vi "Set Page Size.vi"(0 "PDF Report IN":refnum<class "PDF Report Class.lvclass">, 2 "Page setup":T1={"Page Size"=1, "Orientation"=enum."Portrait", "Custom Size"={"Width"=0.0, "Height"=0.0}, "Margins"={"Left"=25.0, "Right"=25.0, "Top"=25.0, "Bottom"=25.0}} {"Page Size" items=["Custom", "LETTER", "NOTE", "LEGAL", "TABLOID", "EXECUTIVE", "POSTCARD", "A0", "A1", "A2", "A3", "A4", "A5", "A6", "A7", "A8", "A9", "A10", "B0", "B1", "B2", "B3", "B4", "B5", "B6", "B7", "B8", "B9", "B10", "ARCH_E", "ARCH_D", "ARCH_C", "ARCH_B", "ARCH_A", "FLSA", "FLSE", "HALFLETTER", "_11X17", "ID_1", "ID_2", "ID_3", "LEDGER", "CROWN_QUARTO", "LARGE_CROWN_QUARTO", "DEMY_QUARTO", "ROYAL_QUARTO", "CROWN_OCTAVO", "LARGE_CROWN_OCTAVO", "DEMY_OCTAVO", "ROYAL_OCTAVO", "SMALL_PAPERBACK", "PENGUIN_SMALL_PAPERBACK", "PENGUIN_LARGE_PAPERBACK"]}, 11 "error in (no error)":errorcluster) -> (4 "PDF Report OUT":refnum<class "PDF Report Class.lvclass">, 15 "error OUT":errorcluster)   [LabVIEW 2019]
doc: "Creates a page break within the PDF report and change the layout of the new page:\n- Page size;\n- Orientation;\n- Margins (mm or in);\n- Custom layout (if Page size = custom, mm or in);\n\nMinimum page size: 3 points x 3 points (1.06 mm x 1.06 mm or 0.042 in x 0.042 in)\nMaximum page size: 14400 points x 14400 points (5.08 m x 5.08 m or 200 in x 200 in)\n\n<B>FRANÇAIS</B>\nAjoute un saut de page dans le rapport PDF et change les caractéristiques de la nouvelle page :\n- Format de la page;\n- Orientation;\n- Marges (mm or in);\n- Format personnalisé (si Page size = custom, mm ou in).\n\nDimensions minimales d'une page: 3 points x 3 points (1.06 mm x 1.06 mm or 0.042 in x 0.042 in).\nDimensions maximales d'une page: 14400 points x 14400 points (5.08 m x 5.08 m or 200 in x 200 in).\n\nVersion 1.0\nDeveloped by Jean-Marc Simard\nCopyright © 2010, Exaprom Inc.\nAll rights reserved.\nLicense: BSD\n\nWith iTextSharp 4.1.6 (http://itextsharp.sourceforge.net)\nunder Mozilla Public License Version 1.1\n(http://www.mozilla.org/MPL/MPL-1.1.html)"
uses:
  <userlib>/Exaprom PDF/Controls/Page Controls/Page setup.ctl
  <userlib>/Exaprom PDF/Controls/Page Controls/Page size.ctl
  <userlib>/Exaprom PDF/Controls/Page Controls/Page Orientation.ctl
  <userlib>/Exaprom PDF/Controls/Page Controls/Page Layout Custom.ctl
  <userlib>/Exaprom PDF/Controls/Page Controls/Page margins.ctl
  <userlib>/Exaprom PDF/LV Class/PDF Report Class/PDF Report Class.lvclass
  C:/Program Files/National Instruments/LabVIEW 2019/user.lib/Exaprom PDF/DLL/itextsharp.dll
  DLL/itextsharp.dll
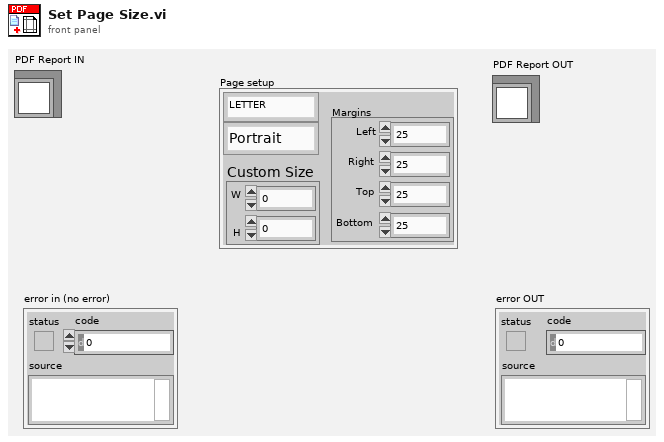
[diagram p1: front panel]
types:
  T1 = typedef "Page setup.ctl" = cluster{"Page Size":T2, "Orientation":T3, "Custom Size":T4, "Margins":T5}
  T2 = typedef "Page size.ctl" = i32
  T3 = typedef "Page Orientation.ctl" = enum16{"Portrait", "Landscape"}
  T4 = typedef "Page Layout Custom.ctl" = cluster{"Width":sgl, "Height":sgl}
  T5 = typedef "Page margins.ctl" = cluster{"Left":sgl, "Right":sgl, "Top":sgl, "Bottom":sgl}
  T6 = typedef "Page dimensions.ctl" = cluster{"Start at page":i32, "Page Size":T2, "Orientation":T3, "widht":sgl, "height":sgl, "Margin left":sgl, "Margin right":sgl, "Margin top":sgl, "Margin bottom":sgl, "X0":sgl, "X1":sgl, "Y0":sgl, "Y1":sgl}
  T7 = typedef "Unit.ctl" = enum16{"inch", "mm"}
  T8 = cluster{"PageNumber":i32, "Page Size":T2, "Orientation":T3, "Width":sgl, "Height":sgl, "LeftMargin":sgl, "RightMargin":sgl, "TopMargin":sgl, "BottomMargin":sgl, "widht":sgl, "Width":sgl, "widht":sgl, "Height":sgl}
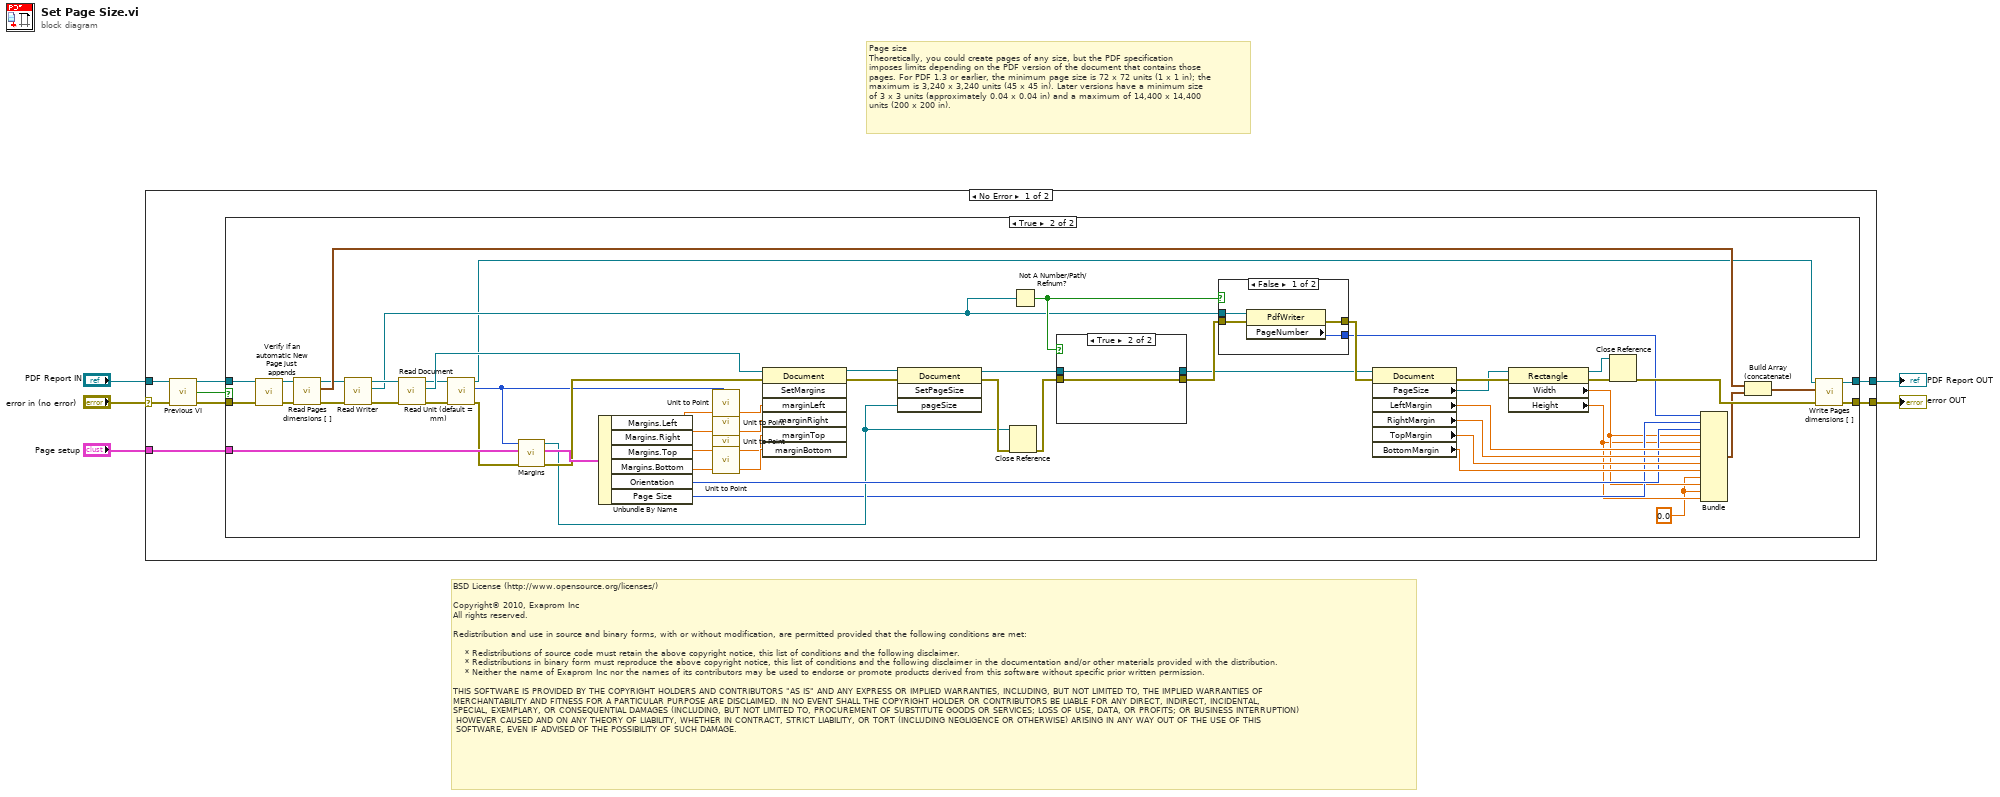
[diagram p0: block diagram]
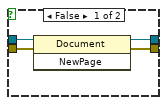
[diagram p3: hidden frame]
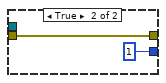
[diagram p4: hidden frame]
diagram:
  # "Page size\nTheoretically, you could create pages of any size, but the PDF specification\nimposes limits depending on the PDF version of the document that contains those\npages. For PDF 1.3 or earlier, the minimum page size is 72 x 72 units (1 x 1 in); the\nmaximum is 3,240 x 3,240 units (45 x 45 in). Later versions have a minimum size\nof 3 x 3 units (approximately 0.04 x 0.04 in) and a maximum of 14,400 x 14,400\nunits (200 x 200 in)."
  # "BSD License (http://www.opensource.org/licenses/)\n\nCopyright© 2010, Exaprom Inc\nAll rights reserved.\n\nRedistribution and use in source and binary forms, with or without modification, are permitted provided that the following conditions are met:\n\n    * Redistributions of source code must retain the above copyright notice, this list of conditions and the following disclaimer.\n    * Redistributions in binary form must reproduce the above copyright notice, this list of conditions and the following disclaimer in the documentation and/or other materials provided with the distribution.\n    * Neither the name of Exaprom Inc nor the names of its contributors may be used to endorse or promote products derived from this software without specific prior written permission.\n\nTHIS SOFTWARE IS PROVIDED BY THE COPYRIGHT HOLDERS AND CONTRIBUTORS \"AS IS\" AND ANY EXPRESS OR IMPLIED WARRANTIES, INCLUDING, BUT NOT LIMITED TO, THE IMPLIED WARRANTIES OF \nMERCHANTABILITY AND FITNESS FOR A PARTICULAR PURPOSE ARE DISCLAIMED. IN NO EVENT SHALL THE COPYRIGHT HOLDER OR CONTRIBUTORS BE LIABLE FOR ANY DIRECT, INDIRECT, INCIDENTAL,\nSPECIAL, EXEMPLARY, OR CONSEQUENTIAL DAMAGES (INCLUDING, BUT NOT LIMITED TO, PROCUREMENT OF SUBSTITUTE GOODS OR SERVICES; LOSS OF USE, DATA, OR PROFITS; OR BUSINESS INTERRUPTION)\n HOWEVER CAUSED AND ON ANY THEORY OF LIABILITY, WHETHER IN CONTRACT, STRICT LIABILITY, OR TORT (INCLUDING NEGLIGENCE OR OTHERWISE) ARISING IN ANY WAY OUT OF THE USE OF THIS\n SOFTWARE, EVEN IF ADVISED OF THE POSSIBILITY OF SUCH DAMAGE."
  n1 = case shown="No Error" "error in (no error)" {
    selector: "error in (no error)" -> [w9 w85]
    tunnel: [w11 w85] -> w3
    tunnel: "Page setup" -> [w6 _]
    tunnel: [w13 w84] -> w2
    tunnel: "PDF Report IN" -> [w12 w84]
    frame No Error {
      n2 = call <userlib>:"Previous VI.vi"("PDF Report IN"=w12, "error in (no error)"=w9) -> ("PDF Report OUT"=w10:refnum<class "PDF Report Class.lvclass">, "Execute Actual VI"=w8:bool, "error out"=w7:errorcluster)  [unwired: 11 out]
      n3 = case shown="True" w8 {
        tunnel: w6 -> [_ w71]
        tunnel: [w14 w23] -> w13
        tunnel: [w15 w25] -> w11
        tunnel: w10 -> [w14 w41]
        tunnel: w7 -> [w15 w38]
        frame False {
        }
        frame True {
          w16 = sgl 0.0 ("widht")
          n4 = call <userlib>:"Verify if an automatic New Page just appends.vi"("PDF Report IN"=w41, "error in (no error)"=w38) -> ("PDF Report OUT"=w39:refnum<class "PDF Report Class.lvclass">, "error out"=w31:errorcluster)  [unwired: 12 out]
          n5 = call-dynamic "Read Pages dimensions [ ].vi"("error in (no error)"=w31, "PDF Report Class in"=w39) -> ("error out"=w34:errorcluster, "Pages dimensions [ ]"=w36:T6[], "PDF Report Class out"=w35:refnum<class "PDF Report Class.lvclass">)  [unwired: 6 in, 1 out]
          n6 = call-dynamic "Read Writer.vi"("error in (no error)"=w34, "PDF Report Class in"=w35) -> ("error out"=w32:errorcluster, "Writer"=w30:refnum<k24>, "PDF Report Class out"=w33:refnum<class "PDF Report Class.lvclass">)  [unwired: 7 in]
          n7 = call-dynamic "Read Document.vi"("error in (no error)"=w32, "PDF Report Class in"=w33) -> ("error out"=w28:errorcluster, "Document"=w29:refnum<k24>, "PDF Report Class out"=w27:refnum<class "PDF Report Class.lvclass">)  [unwired: 7 in]
          n8 = call-dynamic "Read Unit (default = mm).vi"("error in (no error)"=w28, "PDF Report Class in"=w27) -> ("error out"=w21:errorcluster, "Unit (default = mm)"=w26:T7, "PDF Report Class out"=w22:refnum<class "PDF Report Class.lvclass">)  [unwired: 7 in]
          n9 = call <userlib>:"Margins.vi"("error in (no error)"=w21, "Page setup IN"=w71, "Unit (default = mm)"=w26) -> ("error out"=w44:errorcluster, "Page setup OUT"=w46:T1, "Rectangle"=w43:refnum<k24>)  [unwired: 6 out]
          n10 = Unbundle By Name(w46) -> ("Margins.Left"=w70:sgl, "Margins.Right"=w69:sgl, "Margins.Top"=w68:sgl, "Margins.Bottom"=w67:sgl, "Orientation"=w45:T3, "Page Size"=w19:T2)
          n11 = call <userlib>:"Unit to Point.vi"("X unit"=w70, "Unit (default = mm)"=w26) -> ("X point"=w63:sgl)  [unwired: 7 out]
          n12 = call <userlib>:"Unit to Point.vi"("X unit"=w69, "Unit (default = mm)"=w26) -> ("X point"=w64:sgl)  [unwired: 7 out]
          n13 = call <userlib>:"Unit to Point.vi"("X unit"=w68, "Unit (default = mm)"=w26) -> ("X point"=w65:sgl)  [unwired: 7 out]
          n14 = call <userlib>:"Unit to Point.vi"("X unit"=w67, "Unit (default = mm)"=w26) -> ("X point"=w66:sgl)  [unwired: 7 out]
          n15 = invoke class="Document" method="SetMargins"(reference=w29, error in=w44, "marginLeft"=w63, "marginRight"=w64, "marginTop"=w65, "marginBottom"=w66) -> (reference out=w51:refnum<k24>, error out=w40:errorcluster)  [unwired: 1 in, 5 out]
          n16 = invoke class="Document" method="SetPageSize"(reference=w51, error in=w40, "pageSize"=w43) -> (reference out=w50:refnum<k24>, error out=w57:errorcluster)  [unwired: 1 in, 2 out]
          n17 = Close Reference(reference=w43, error in (no error)=w57) -> (error out=w49:errorcluster)
          n18 = Not A Number/Path/Refnum?(number/path/refnum=w30) -> (NaN/Path/Refnum?=w47:bool)
          n19 = case shown="True" w47 {
            tunnel: [w75 w77] -> w37
            tunnel: [w74 w76] -> w48
            tunnel: w49 -> [w73 w76]
            tunnel: w50 -> [w72 w77]
            frame False {
              n20 = invoke class="Document" method="NewPage"(reference=w72, error in=w73) -> (reference out=w75:refnum<k24>, error out=w74:errorcluster)  [unwired: 1 in, 1 out]
            }
            frame True {
            }
          }
          n21 = case shown="False" w47 {
            tunnel: [w80 1 ("PageNumber")] -> w20
            tunnel: w30 -> [w81 _]
            tunnel: w48 -> [w79 w82]
            tunnel: [w78 w82] -> w52
            frame False {
              n22 = property class="PdfWriter"(reference=w81, error in=w79) -> (error out=w78:errorcluster, "PageNumber"=w80:i32)  [unwired: 1 out]
            }
            frame True {
            }
          }
          n23 = property class="Document"(reference=w37, error in=w52) -> (error out=w62:errorcluster, "PageSize"=w42:refnum<k24>, "LeftMargin"=w61:sgl, "RightMargin"=w60:sgl, "TopMargin"=w59:sgl, "BottomMargin"=w58:sgl)  [unwired: 1 out]
          n24 = property class="Rectangle"(reference=w42, error in=w62) -> (reference out=w55:refnum<k24>, error out=w56:errorcluster, "Width"=w18:sgl, "Height"=w17:sgl)
          n25 = Close Reference(reference=w55, error in (no error)=w56) -> (error out=w54:errorcluster)
          n26 = Bundle("PageNumber"=w20, "Page Size"=w19, "Orientation"=w45, "Width"=w18, "Height"=w17, "LeftMargin"=w61, "RightMargin"=w60, "TopMargin"=w59, "BottomMargin"=w58, "widht"=w16, "Width"=w18, "widht"=w16, "Height"=w17) -> (w53:T8)  [unwired: 1 out]
          n27 = Build Array (concatenate)(w36, w53) -> (w24:T6[])
          n28 = call-dynamic "Write Pages dimensions [ ].vi"("error in (no error)"=w54, "Pages dimensions [ ]"=w24, "PDF Report Class in"=w22) -> ("error out"=w25:errorcluster, "PDF Report Class out"=w23:refnum<class "PDF Report Class.lvclass">)  [unwired: 7 in]
        }
      }
    }
    frame Error {
    }
  }
  "error OUT" <- w3
  "PDF Report OUT" <- w2
